vi "Connect Information.vi"() -> (2 "Connect Info":string)   [LabVIEW 2023]
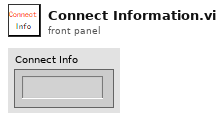
[diagram p1: front panel]
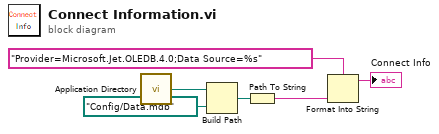
[diagram p0: block diagram]
diagram:
  n1 = call <vilib>:"Application Directory.vi"() -> ("Application Directory"=w5:path)
  n2 = Build Path(base path=w5, name or relative path=path "Config/Data.mdb" ("名称或相对路径")) -> (appended path=w3:path)
  n3 = Path To String(path=w3) -> (string=w2:string)
  n4 = Format Into String(format string="Provider=Microsoft.Jet.OLEDB.4.0;Data Source=%s", w2) -> (resulting string=→"Connect Info":string)  [unwired: 2 in, 1 out]
